vi "SECoP-addWritableParameter.vi"(6 "description":string, 7 "datainfo":string, 8 "error in (no error)":errorcluster, 10 "parameter name":string, 11 "DLL path (in)":T1) -> (0 "error out":errorcluster, 3 "DLL path (out)":T1)   [LabVIEW 2023, in "SECoP.lvlib"]
doc: "Call <b>\"SECoP-addWritableParameter.vi\"</b> to create a read- and writable SECoP parameter inside the last created SECoP module.\n\n<b>DLL path</b> input and output of cluster from \"SECoP-Initialize.vi\"\n<b>parameter name</b> name of parameter\n<b>datainfo</b> data info (data type of parameter, see SECoP specification)\n<b>description</b> human readable description of this parameter"
uses:
  SECoP.lvlib
  SECoP-libraries.ctl
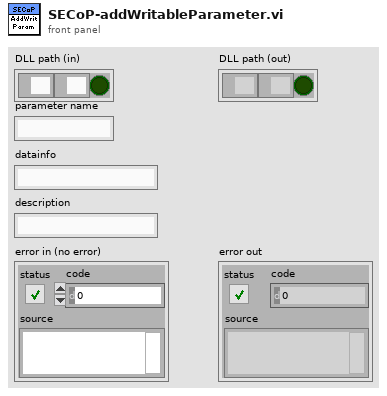
[diagram p1: front panel]
types:
  T1 = typedef "SECoP.lvlib/SECoP-libraries.ctl" = cluster{"serverDLL":path, "variantDLL":path, "cleanup_mode":bool}
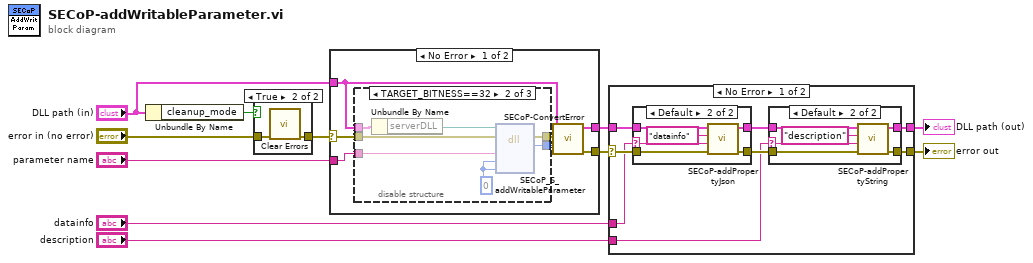
[diagram p0: block diagram]
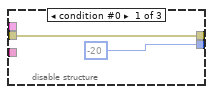
[diagram p6: hidden frame]
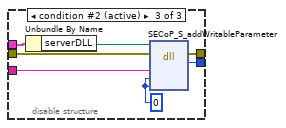
[diagram p7: hidden frame]
diagram:
  n1 = Unbundle By Name("DLL path (in)") -> ("cleanup_mode"=w10:bool)
  n2 = case shown="True" w10 {
    tunnel: "error in (no error)" -> [w12 w14]
    tunnel: [w12 w13] -> w8
    frame False {
    }
    frame True {
      n3 = call <vilib>:"Clear Errors.vi"("error in (no error)"=w14) -> ("error out"=w13:errorcluster)  [unwired: 5 in, 1 out]
    }
  }
  n4 = case shown="No Error" w8 {
    selector: w8 -> [w19 w38]
    tunnel: "DLL path (in)" -> [w15 w39]
    tunnel: [w20 w39] -> w3
    tunnel: [w21 w38] -> w4
    tunnel: "parameter name" -> [w18 _]
    frame No Error {
      n5 = disable-structure shown="TARGET_BITNESS==32" {
        disable-tunnel: w19 -> [w23 w30 w37]
        disable-tunnel: w15 -> [_ w29 w36]
        disable-tunnel: w18 -> [_ w28 w35]
        disable-tunnel: [w23 w26 w33] -> w17
        disable-tunnel: [-20 ("return type") w25 w32] -> w16
        frame condition #0 {
        }
        frame condition #1 {
          w27 = u32 0 ("function pointer (0)")
          n6 = Unbundle By Name(w29) -> ("serverDLL"=w24:path)
          n7 = dll-call lib="C:/Users/user/Desktop/x86_64/SECoP64.dll" fn="SECoP_S_addWritableParameter"(path in=w24, error in=w30, "name"=w28, "function pointer get (0)"=w27, "function pointer set (0)"=w27) -> (error out=w26:errorcluster, "return type"=w25:i32)  [unwired: 4 in, 1 out]
        }
        frame condition #2 (active) {
          w34 = u64 0 ("function pointer (0)")
          n8 = Unbundle By Name(w36) -> ("serverDLL"=w31:path)
          n9 = dll-call lib="C:/Users/user/Desktop/x86_64/SECoP64.dll" fn="SECoP_S_addWritableParameter"(path in=w31, error in=w37, "name"=w35, "function pointer get (0)"=w34, "function pointer set (0)"=w34) -> (error out=w33:errorcluster, "return type"=w32:i32)  [unwired: 4 in, 1 out]
        }
      }
      n10 = call "SECoP-ConvertError.vi"("return code"=w16, "error in (no error)"=w17, "DLL path (in)"=w15) -> ("error out"=w21:errorcluster, "DLL path (out)"=w20:T1)  [unwired: 7 in]
    }
    frame Error {
    }
  }
  n11 = case shown="No Error" w4 {
    selector: w4 -> [w45 w65]
    tunnel: w3 -> [w46 w64]
    tunnel: [w40 w65] -> w1
    tunnel: [w41 w64] -> w2
    tunnel: "datainfo" -> [w44 _]
    tunnel: "description" -> [w43 _]
    frame No Error {
      n12 = case shown="Default" w44 {
        selector: w44 -> [_ w59]
        tunnel: w46 -> [w57 w63]
        tunnel: w45 -> [w56 w62]
        tunnel: [w56 w61] -> w47
        tunnel: [w57 w60] -> w42
        frame "" {
        }
        frame Default {
          n13 = call "SECoP-addPropertyJson.vi"("error in (no error)"=w62, "property value"=w59, "property name"="datainfo", "DLL path (in)"=w63) -> ("error out"=w61:errorcluster, "DLL path (out)"=w60:T1)  [unwired: 6 in]
        }
      }
      n14 = case shown="Default" w43 {
        selector: w43 -> [_ w51]
        tunnel: w42 -> [w49 w55]
        tunnel: w47 -> [w48 w54]
        tunnel: [w48 w53] -> w40
        tunnel: [w49 w52] -> w41
        frame "" {
        }
        frame Default {
          n15 = call "SECoP-addPropertyString.vi"("error in (no error)"=w54, "property value"=w51, "property name"="description", "DLL path (in)"=w55) -> ("error out"=w53:errorcluster, "DLL path (out)"=w52:T1)  [unwired: 6 in]
        }
      }
    }
    frame Error {
    }
  }
  "DLL path (out)" <- w2
  "error out" <- w1
